vi "Write_control.vi"(8 "error in (no error)":errorcluster, 9 "data":variant, 10 "control_label":string="stop", 11 "VI ref in":refnum<vi>) -> (0 "error out":errorcluster, 3 "ref out":refnum<vi>)   [LabVIEW 2012]
doc: "Записывает данные в управляющий элемент (control) по его метке (Lable)"
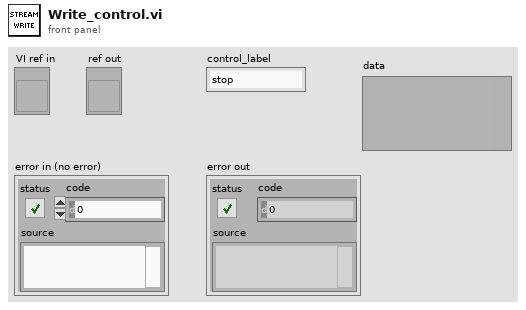
[diagram p1: front panel]
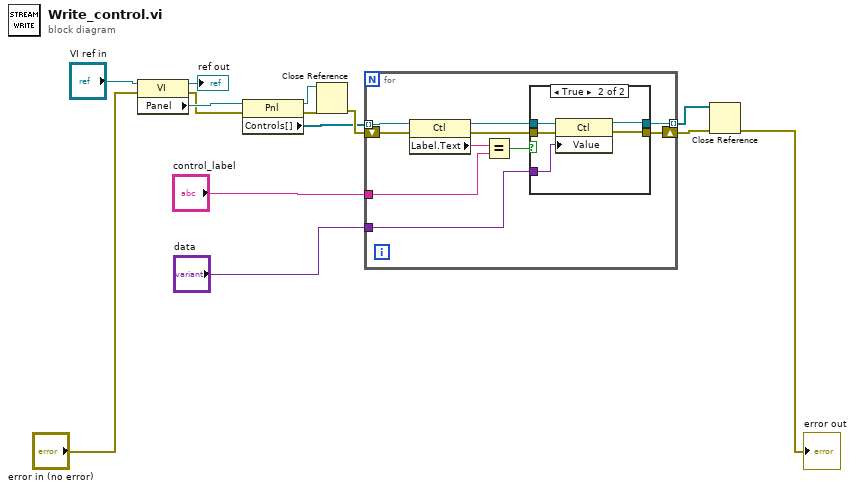
[diagram p0: block diagram]
diagram:
  n1 = property class="VI"(reference="VI ref in", error in="error in (no error)") -> (reference out=→"ref out":refnum<vi>, error out=w2:errorcluster, "Panel"=w11:refnum<vi>)
  n2 = property class="Pnl"(reference=w11, error in=w2) -> (reference out=w13:refnum<vi>, error out=w12:errorcluster, "Controls[]"=w5:refnum<vi>[])
  n3 = Close Reference(reference=w13, error in (no error)=w12) -> (error out=w14:errorcluster)
  n4 = for {
    tunnel: w5 -> [w24] mode=indexing
    tunnel: "control_label" -> [w22]
    tunnel: [w18] -> w8 mode=indexing
    tunnel: "data" -> [w16]
    shift-right: [w17] -> w9
    shift-left: w14 -> [w15]
    n5 = property class="Ctl"(reference=w24, error in=w15) -> (reference out=w21:refnum<vi>, error out=w20:errorcluster, "Label.Text"=w23:string)
    n6 = Equal?(x=w23, y=w22) -> (x = y?=w19:bool)
    n7 = case shown="True" w19 {
      tunnel: w21 -> [w26 w31]
      tunnel: w20 -> [w25 w30]
      tunnel: [w26 w28] -> w18
      tunnel: [w25 w29] -> w17
      tunnel: w16 -> [_ w27]
      frame False {
      }
      frame True {
        n8 = property class="Ctl"(reference=w31, error in=w30, "Value"=w27) -> (reference out=w28:refnum<vi>, error out=w29:errorcluster)
      }
    }
  }
  n9 = Close Reference(reference=w8, error in (no error)=w9) -> (error out=→"error out":errorcluster)
